vi "RunAcquisition.vi"(8 "error in (no error)":errorcluster, 11 "IVI_Class in":refnum<class "IVI_Class.lvclass">) -> (0 "error out":errorcluster, 2 "Waveforms":T1[](array[typedef]), 3 "IVI_Class out":refnum<class "IVI_Class.lvclass">)   [LabVIEW 2018, in "ScopePlugins.lvlib" / "IVI_Class.lvclass"]
uses:
  IVI_Class.lvclass
  C:/Users/ico/Documents/Projects/NistPluggableModules/Scope/ScopePlugins/ScopePluginBaseClass/ScopePluginsBase.lvclass
  ScopeShared/Waveform.ctl
  ScopePluginBaseClass/ScopePluginsBase.lvclass/ScopePluginsBase.ctl
  ScopePluginBaseClass/Accessors/Read Handle.vi
  ScopePluginBaseClass/Accessors/Read Acquisition.vi
  ScopePluginBaseClass/Accessors/Read Channels.vi
  ScopePluginBaseClass/Accessors/Read Connected.vi
  <vilib>/Utility/error.llb/Error Cluster From Error Code.vi
  <vilib>/ErrorRing/Error Ring.xnode
  ScopeShared/ScopeShared.lvlib
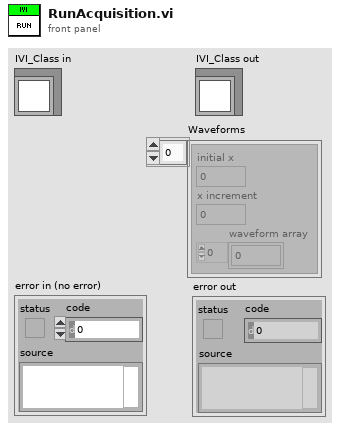
[diagram p1: front panel]
types:
  T1 = typedef "ScopeShared.lvlib/Waveform.ctl" = cluster{"initial x":dbl, "x increment":dbl, "waveform array":dbl[]}
  T2 = cluster{"initial x":dbl, "x increment":dbl, "waveform array":dbl[]}[]
  T3 = typedef "ScopePlugins.lvlib/Acquisition.ctl" = cluster{"StartTime":dbl, "Type":enum16{"Normal", "PeakDetect", "HighRes", "Envelope", "Average"}, "NumPointsMin":i32, "RecordLength":i32, "SampleRate":dbl, "TimePerRecord":dbl, "SamplingMode ":enum16{"Real Time", "Equivalent Time", "Segment", "Real Time Peak Detect", "Real Time High Resolution", "Peak Detect Segment", "High Resolution Segment"}, "Interpolation":enum16{"No Interpolation", "sin(x)/x", "linear", "1 Point sin(x)/x", "2 Point sin(x)/x", "4 Point sin(x)/x", "8 Point sin(x)/x", "16 Point sin(x)/x"}, "NumAverages":i32, "Resolution":enum16{"Auto", "Bits 9", "Bits 10", "Bits 11", "Bits 12"}, "EnableAveraging":bool, "Continuous":bool}
  T4 = typedef "ScopePlugins.lvlib/Channels.ctl" = cluster{"Count":i32, "ChannelArray":T5[]}
  T5 = typedef "ScopePlugins.lvlib/Channel.ctl" = cluster{"Enabled":bool, "Name":string, "InputImpedance":dbl, "InputFreqMax":dbl, "ProbeAttn":dbl, "Coupling":enum16{"AC", "DC", "GND"}, "Offset":dbl, "Range":dbl, "Handle":string, "Connected":bool, "Options String ":string}
  T6 = cluster{"initial x":dbl, "x increment":dbl, "waveform array":dbl[]}
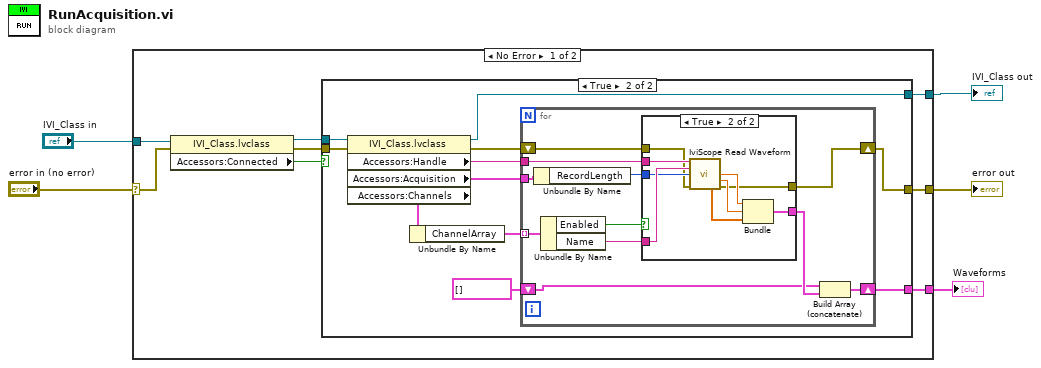
[diagram p0: block diagram]
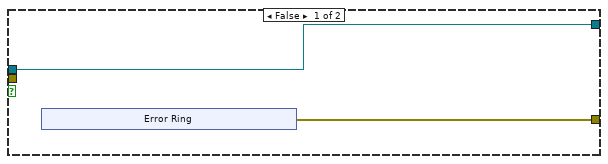
[diagram p2: hidden frame]
diagram:
  n1 = case shown="No Error" "error in (no error)" {
    selector: "error in (no error)" -> [w12 w53]
    tunnel: "IVI_Class in" -> [w13 w54]
    tunnel: [w8 w54] -> w3
    tunnel: [w9 w53] -> w2
    tunnel: [w6 _] -> w1
    frame No Error {
      n2 = property class="IVI_Class.lvclass"(reference=w13, error in=w12) -> (reference out=w10:refnum<class "IVI_Class.lvclass">, error out=w7:errorcluster, "Accessors:Connected"=w11:bool)
      n3 = case shown="True" w11 {
        tunnel: w10 -> [w14 w31]
        tunnel: [w15 w23] -> w9
        tunnel: [w14 w22] -> w8
        tunnel: w7 -> [_ w30]
        tunnel: [_ w24] -> w6
        frame False {
          n4 = xnode "Error Ring"() -> ("error out"=w15:errorcluster)
        }
        frame True {
          n5 = property class="IVI_Class.lvclass"(reference=w31, error in=w30) -> (reference out=w22:refnum<class "IVI_Class.lvclass">, error out=w25:errorcluster, "Accessors:Handle"=w29:string, "Accessors:Acquisition"=w26:T3, "Accessors:Channels"=w28:T4)
          n6 = Unbundle By Name(w28) -> ("ChannelArray"=w27:T5[])
          n7 = for {
            tunnel: w29 -> [w42]
            tunnel: w27 -> [w41] mode=indexing
            tunnel: w26 -> [w38]
            shift-right: [w34] -> w24
            shift-left: T2 [] -> [w33]
            shift-right: [w32] -> w23
            shift-left: w25 -> [w36]
            n8 = Unbundle By Name(w38) -> ("RecordLength"=w37:i32)
            n9 = Unbundle By Name(w41) -> ("Enabled"=w40:bool, "Name"=w39:string)
            n10 = case shown="True" w40 {
              tunnel: w42 -> [_ w52]
              tunnel: w39 -> [_ w51]
              tunnel: w37 -> [_ w50]
              tunnel: w36 -> [w43 w49]
              tunnel: [w43 w45] -> w32
              tunnel: [_ w44] -> w35
              frame False {
              }
              frame True {
                n11 = call <vilib>:"IviScope Read Waveform.vi"("instrument handle"=w52, "channel name (\"CHANNEL1\")"=w51, "waveform size (0)"=w50, "error in (no error)"=w49) -> ("initial x"=w48:dbl, "x increment"=w47:dbl, "waveform array"=w46:dbl[], "error out"=w45:errorcluster)  [unwired: 6 in, 2 out]
                n12 = Bundle("initial x"=w48, "x increment"=w47, "waveform array"=w46) -> (w44:T6)  [unwired: 1 out]
              }
            }
            n13 = Build Array (concatenate)(w33, w35) -> (w34:T2)
          }
        }
      }
    }
    frame Error {
    }
  }
  "error out" <- w2
  "IVI_Class out" <- w3
  "Waveforms" <- w1
